vi "VIS-IR_INIT_drv.vi"(8 "error in (no error)":errorcluster, 11 "VIS-IR in":refnum<class "VIS-IR.lvclass">) -> (0 "error out":errorcluster, 3 "Detector out":refnum<class "VIS-IR.lvclass">)   [LabVIEW 2015, in "Detector.lvclass"]
uses:
  Detector.lvclass
  VIS-IR.lvclass
  dependecies/ControlsVIs/Clusters-def/list-of-DAQmx-tasks.ctl
  dependecies/ControlsVIs/Clusters-def/list-of-keys-DAQmx-tasks.ctl
  GeneralFunctionality/GeneralFunctionality.lvclass/GeneralFunctionality.ctl
  Detector.lvclass/Detector.ctl
  dependecies/globalVarII.vi
  Config/Config.lvclass
  GeneralFunctionality/GeneralFunctionality.lvclass
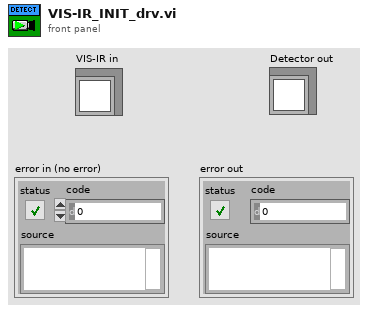
[diagram p1: front panel]
types:
  T1 = typedef "list-of-keys-DAQmx-tasks.ctl" = string
  T2 = typedef "list-of-DAQmx-tasks.ctl" = string
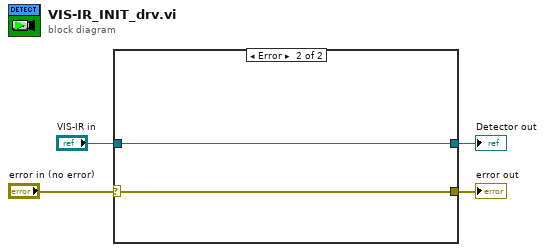
[diagram p0: block diagram]
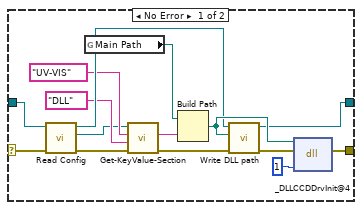
[diagram p2: hidden frame]
diagram:
  n1 = case shown="Error" "error in (no error)" {
    selector: "error in (no error)" -> [w5 w20]
    tunnel: [w18 w20] -> w4
    tunnel: "VIS-IR in" -> [w7 w21]
    tunnel: [w6 w21] -> w2
    frame No Error {
      n2 = call "Read Config.vi"("error in (no error)"=w5, "GeneralFunctionality en entrée"=w7) -> ("error out"=w9:errorcluster, "Config.lvclass"=w11:refnum<class "Config.lvclass">, "GeneralFunctionality en sortie"=w17:refnum<class "VIS-IR.lvclass">)  [unwired: 7 in]
      n3 = global read "globalVarII.vi" "Main Path"() -> (w12:path)
      n4 = call-dynamic "Get-KeyValue-Section.vi"("error in (no error)"=w9, "Key"=T1 "DLL", "Section"=T2 "UV-VIS", "Config in"=w11) -> ("error out"=w10:errorcluster, "Value"=w13:string)  [unwired: 5 in, 1 out]
      n5 = Build Path(base path=w12, name or relative path=w13) -> (appended path=w19:path)
      n6 = call "Write DLL path.vi"("error in (no error)"=w10, "DLL path"=w19, "Detector in"=w17) -> ("error out"=w16:errorcluster, "Detector out"=w6:refnum<class "VIS-IR.lvclass">)  [unwired: 7 in]
      n7 = dll-call lib="C:/Users/Sergey Denisov/Desktop/TRANCON/DLL/ESLSCDLL.dll" fn="_DLLCCDDrvInit@4" ("lwlscdll.dll:DLLCCDDrvInit")(path in=w19, error in=w16, "drv"=u32 1) -> (error out=w18:errorcluster)  [unwired: 3 in, 1 out]
    }
    frame Error {
    }
  }
  "error out" <- w4
  "Detector out" <- w2
